vi "二值化阈值自动调节（灰度版）.vi"(1 "控制黑白百分比（0-100）默认100":dbl, 2 "输入image数组（灰度）":dbl[][](array[numeric])) -> (0 "二值化阈值":dbl)   [LabVIEW 2017]
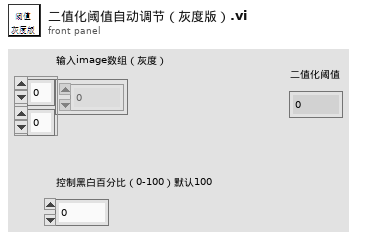
[diagram p1: front panel]
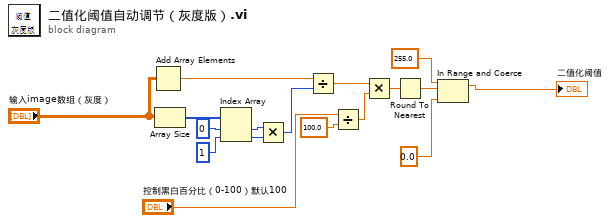
[diagram p0: block diagram]
diagram:
  n1 = Add Array Elements(numeric array="输入image数组（灰度）") -> (sum=w12:dbl)
  n2 = Array Size(array="输入image数组（灰度）") -> (size(s)=w17:i32[])
  n3 = Index Array(array=w17, index #1=0, index #2=1) -> (element #1=w14:i32, element #2=w13:i32)
  n4 = Multiply(x=w14, y=w13) -> (x*y=w10:i32)
  n5 = Divide(x=w12, y=w10) -> (x/y=w6:dbl)
  n6 = Divide(x="控制黑白百分比（0-100）默认100", y=100.0) -> (x/y=w7:dbl)
  n7 = Multiply(x=w6, y=w7) -> (x*y=w5:dbl)
  n8 = Round To Nearest(number=w5) -> (nearest integer value=w4:dbl)
  n9 = In Range and Coerce(upper limit=255.0, x=w4, lower limit=0.0) -> (coerced(x)=→"二值化阈值":dbl)  [unwired: 1 out]
